vi "WireWriteBlockDiagram.vi"(8 "error in":errorcluster, 10 "Terminal References":T4, 11 "State":T1) -> (0 "error out":errorcluster, 3 "State out":T1)   [LabVIEW 2013, in "data interface script.lvlib"]
uses:
  data interface script.lvlib
  Controls/TerminalReferences.ctl
  Controls/StateCluster.ctl
  Controls/initialized references.ctl
  Controls/interface VI type.ctl
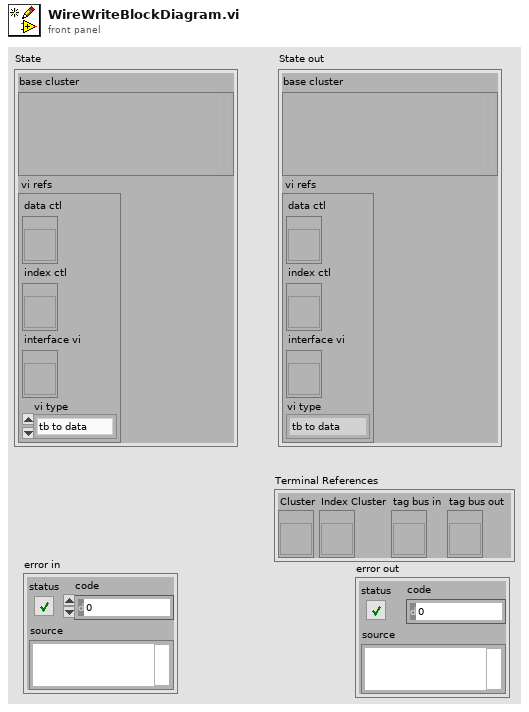
[diagram p1: front panel]
types:
  T1 = typedef "data interface script.lvlib/StateCluster.ctl" = cluster{"base cluster":variant, "vi refs":T2}
  T2 = typedef "data interface script.lvlib/initialized references.ctl" = cluster{"data ctl":refnum<vi>, "index ctl":refnum<vi>, "interface vi":refnum<vi>, "vi type":T3}
  T3 = typedef "data interface script.lvlib/interface VI type.ctl" = enum16{"tb to data", "data to tb"}
  T4 = typedef "data interface script.lvlib/TerminalReferences.ctl" = cluster{"Cluster":refnum<vi>, "Index Cluster":refnum<vi>, "tag bus in":refnum<vi>, "tag bus out":refnum<vi>}
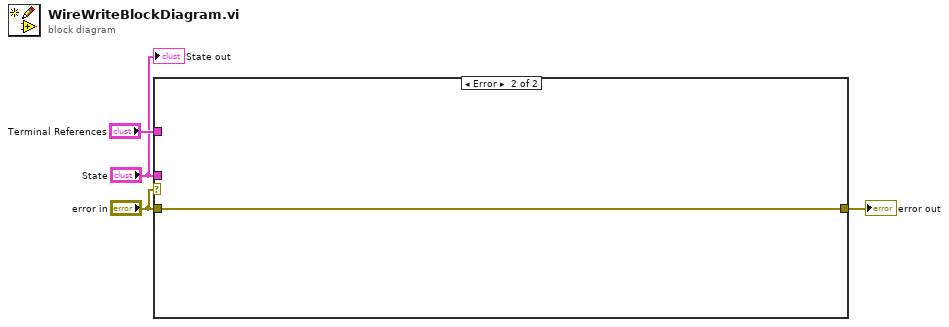
[diagram p0: block diagram]
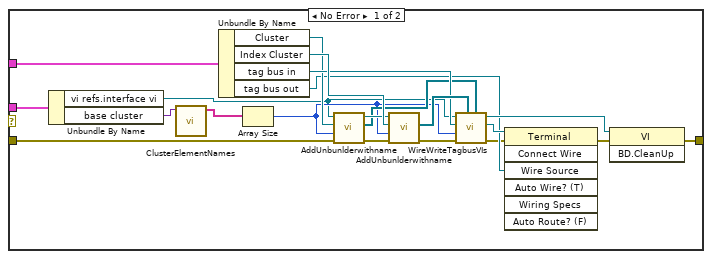
[diagram p2: hidden frame]
diagram:
  n1 = case shown="Error" "error in" {
    tunnel: "Terminal References" -> [w25 _]
    tunnel: [w24 w26] -> w3
    tunnel: "State" -> [w19 _]
    tunnel: "error in" -> [w17 w26]
    frame No Error {
      n2 = Unbundle By Name(w19) -> ("vi refs.interface vi"=w6:refnum<vi>, "base cluster"=w21:variant)
      n3 = call "ClusterElementNames.vi"("input cluster"=w21) -> ("Elements Names"=w20:string[])  [unwired: 8 in, 2 out]
      n4 = Unbundle By Name(w25) -> ("Cluster"=w16:refnum<vi>, "Index Cluster"=w23:refnum<vi>, "tag bus in"=w18:refnum<vi>, "tag bus out"=w10:refnum<vi>)
      n5 = Array Size(array=w20) -> (size(s)=w7:i32)
      n6 = call "AddUnbunlderwithname.vi"("error in"=w17, "elements in cluster"=w7, "cluster terminal"=w16, "VI in"=w6) -> ("error out"=w14:errorcluster, "terminals"=w8:refnum<vi>[], "VI out"=w15:refnum<vi>)  [unwired: 5 in]
      n7 = call "AddUnbunlderwithname.vi"("error in"=w14, "elements in cluster"=w7, "cluster terminal"=w23, "VI in"=w15) -> ("error out"=w9:errorcluster, "terminals"=w22:refnum<vi>[])  [unwired: 5 in, 1 out]
      n8 = call "WireWriteTagbusVIs.vi"("terminals data"=w8, "terminals indexes"=w22, "error in"=w9, "elements in cluster"=w7, "tag bus in in"=w18, "VI in"=w6) -> ("error out"=w5:errorcluster, "tag bus out"=w11:refnum<vi>, "VI out"=w13:refnum<vi>)  [unwired: 3 in]
      n9 = invoke on="Invoke Node" class="Terminal" method="Connect Wire"(reference=w11, error in=w5, "Wire Source"=w10) -> (error out=w12:errorcluster)  [unwired: 4 in, 6 out]
      n10 = invoke class="VI" method="BD.CleanUp"(reference=w13, error in=w12) -> (error out=w24:errorcluster)  [unwired: 1 in, 2 out]
    }
    frame Error {
    }
  }
  "error out" <- w3
  "State out" <- "State"
